vi "WSVCAP SHL FPGA LL Procedure I2C - Send ACK.vi"(0 "Procedure Step":T1, 1 "Wait Ticks Remaining":u32, 5 "I2C Wait Ticks":u32, 7 "ACK Bit to Write":bool, 11 "error in (no error)":errorcluster, 13 "Socket Mask":u64 format="%012x", 14 "UUT (0/1)":u8) -> (3 "Wait Ticks Remaining Out":u32, 4 "Procedure Step Out":T1, 8 "Finished":bool, 15 "error out":errorcluster)   [LabVIEW 2017]
uses:
  Type Defs/WSVCAP SHL Procedure Step Enum.ctl
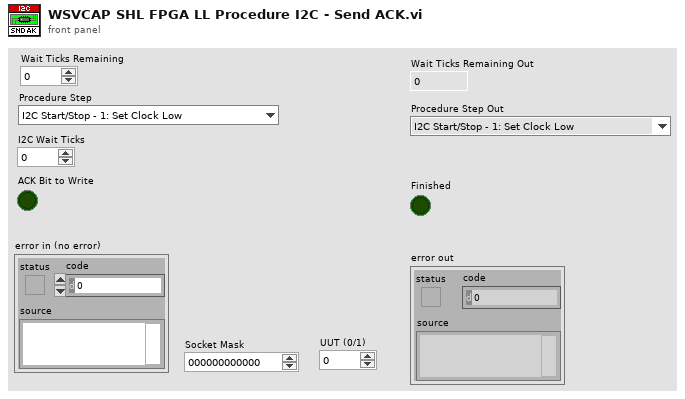
[diagram p1: front panel]
types:
  T1 = typedef "WSVCAP SHL Procedure Step Enum.ctl" = enum16{"I2C Start/Stop - 1: Set Clock Low", "I2C Start/Stop - 2: Wait", "I2C Start/Stop - 3: Set Data I", "I2C Start/Stop - 4: Wait", "I2C Start/Stop - 5: Set Clock High", "I2C Start/Stop - 6: Wait", "I2C Start/Stop - 7: Set Data II", "I2C Start/Stop - 8: Wait", "I2C Start/Stop - 9: Set Clock Low", "I2C Start/Stop - 10: Wait", "I2C Read ACK - 1: Set Clock High", "I2C Read ACK - 2: Wait", "I2C Read ACK - 3: Read ACK Bit", "I2C Read ACK - 4: Wait", "I2C Read ACK - 5: Set Clock Low", "I2C Read ACK - 6: Wait", "I2C Write ACK - 1: Write ACK Bit", "I2C Write ACK - 2: Wait", "I2C Write ACK - 3: Set Clock High", "I2C Write ACK - 4: Wait", "I2C Write ACK - 5: Set Clock Low", "I2C Write ACK - 6: Wait", "I2C Write ACK - 7: Set Data Low", "I2C Send Add - 1: Reset Bits Remaining", "I2C Send Add - 2: Set Data Bit", "I2C Send Add - 3: Wait", "I2C Send Add - 4: Set Clock High", "I2C Send Add - 5: Wait", "I2C Send Add - 6: Set Clock Low", "I2C Send Add - 7: Wait", "I2C Send Add - 8: Check Bits Remaining", "I2C Send Data - 1: Reset Bits Remaining", "I2C Send Data - 2: Load Write Bit from FIFO", "I2C Send Data - 3: Set Data Bit", "I2C Send Data - 4: Wait", "I2C Send Data - 5: Set Clock High", "I2C Send Data - 6: Wait", "I2C Send Data - 7: Set Clock Low", "I2C Send Data - 8: Wait", "I2C Send Data - 9: Check Bits Remaining", "I2C Receive Data - 1: Reset Bits Remaining", "I2C Receive Data - 2: Wait", "I2C Receive Data - 3: Set Clock High", "I2C Receive Data - 4: Wait", "I2C Receive Data - 5: Read Data Bit", "I2C Receive Data - 6: Wait", "I2C Receive Data - 7: Set Clock Low", "I2C Receive Data - 8: Wait", "I2C Receive Data - 9: Check Bits Remaining", "RFFE Send SSC - 1:Set Low", "RFFE Send SSC - 2:Wait", "RFFE Send SSC - 3:Set SDA High", "RFFE Send SSC - 4:Wait", "RFFE Send SSC - 5:Set SDA Low", "RFFE Send SSC - 6:Wait", "RFFE Send Data - 1:Set SCL High", "RFFE Send Data - 2:Wait", "RFFE Send Data - 3:Set SCL Low", "RFFE Send Data - 4:Wait", "RFFE Send Data - 5:Set SCL High (P)", "RFFE Send Data - 6:Wait", "RFFE Send Data - 7:Set SCL Low (P)", "RFFE Send Data - 8:Wait", "RFFE Send Data - 9:Set SCL High (BP)", "RFFE Send Data - 10:Wait", "RFFE Send Data - 11:Set SCL Low (BP)", "RFFE Send Data - 12:Wait", "RFFE Receive Data - 1:Set SCL High", "RFFE Receive Data - 2:Wait", "RFFE Receive Data - 3:Set SCL Low", "RFFE Receive Data - 4:Wait", "RFFE Receive Data - 5:Set SCL High (BP)", "RFFE Receive Data - 6:Wait", "RFFE Receive Data - 7:Set SCL Low (BP)", "RFFE Receive Data - 8:Wait", "RFFE Wait CMD Delay - 1:Wait", "RFFE Clear Lines - 1:Clear"}
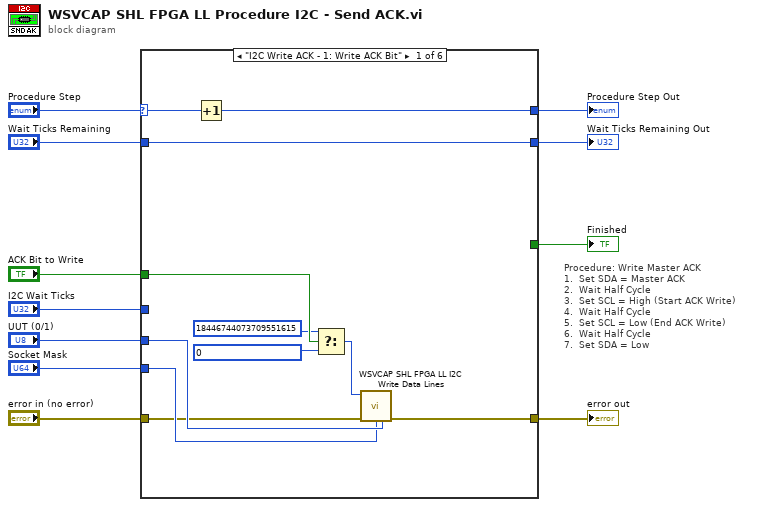
[diagram p0: block diagram]
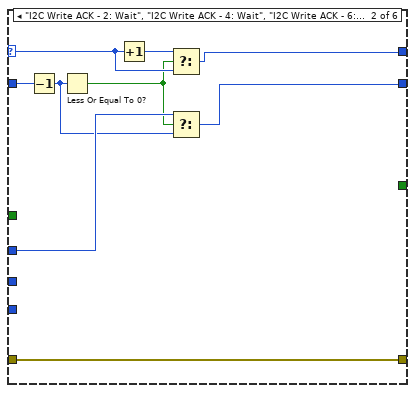
[diagram p2: hidden frame]
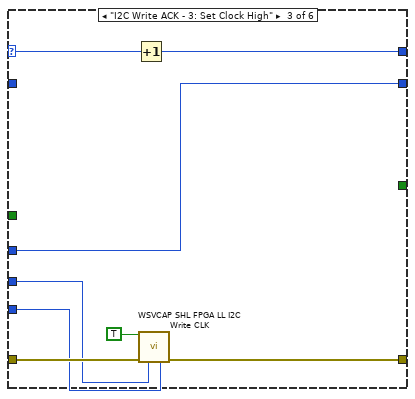
[diagram p3: hidden frame]
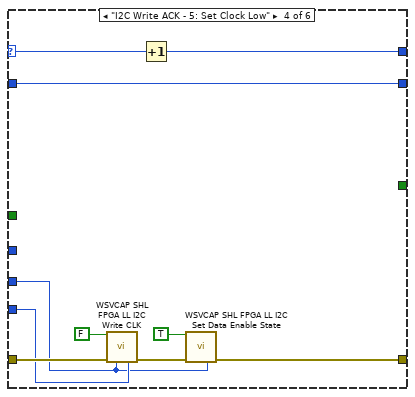
[diagram p4: hidden frame]
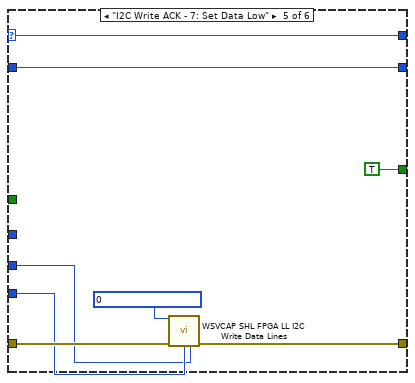
[diagram p5: hidden frame]
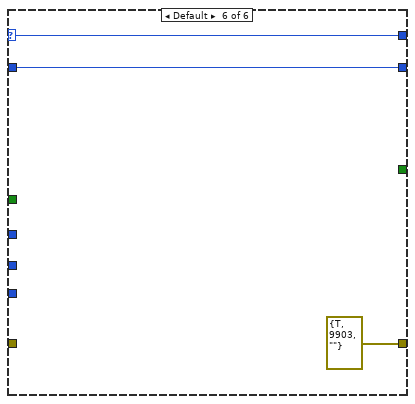
[diagram p6: hidden frame]
diagram:
  # "Procedure: Write Master ACK\n1.  Set SDA = Master ACK\n2.  Wait Half Cycle\n3.  Set SCL = High (Start ACK Write)\n4.  Wait Half Cycle\n5.  Set SCL = Low (End ACK Write)\n6.  Wait Half Cycle\n7.  Set SDA = Low"
  n1 = case shown="\"I2C Write ACK - 1: Write ACK Bit\"" "Procedure Step" {
    selector: "Procedure Step" -> [w22 w26 w37 w44 w56 w59]
    tunnel: [w19 w29 w36 w46 w52 errorcluster {"status"=TRUE, "code"=9903, "source"=""} ("error out")] -> w10
    tunnel: "error in (no error)" -> [w12 w29 w39 w49 w53 _]
    tunnel: "Wait Ticks Remaining" -> [w20 w31 _ w41 w55 w58]
    tunnel: "I2C Wait Ticks" -> [_ w28 w33 _ _ _]
    tunnel: [_ _ _ _ TRUE _] -> w9
    tunnel: "ACK Bit to Write" -> [w18 _ _ _ _ _]
    tunnel: "Socket Mask" -> [w13 _ w35 w43 w51 _]
    tunnel: [w21 w24 w34 w42 w56 w59] -> w3
    tunnel: [w20 w23 w33 w41 w55 w58] -> w2
    tunnel: "UUT (0/1)" -> [w14 _ w32 w40 w50 _]
    frame "I2C Write ACK - 1: Write ACK Bit" {
      n2 = Increment(x=w22) -> (x+1=w21:T1)
      n3 = Select(t=u64 18446744073709551615 ("Write Bit (U64)"), s=w18, f=u64 0 ("Write Bit (U64)")) -> (s? t:f=w15:u64)
      n4 = call "WSVCAP SHL FPGA LL I2C Write Data Lines.vi"("Write Bit (U64)"=w15, "error in (no error)"=w12, "Socket Mask"=w13, "UUT Set (0/1) (Legacy)"=w14) -> ("error out"=w19:errorcluster)  [unwired: 11 in]
    }
    frame "I2C Write ACK - 2: Wait", "I2C Write ACK - 4: Wait", "I2C Write ACK - 6: Wait" {
      n5 = Decrement(x=w31) -> (x-1=w27:u32)
      n6 = Less Or Equal To 0?(x=w27) -> (x <= 0?=w25:bool)
      n7 = Increment(x=w26) -> (x+1=w30:T1)
      n8 = Select(t=w30, s=w25, f=w26) -> (s? t:f=w24:T1)
      n9 = Select(t=w28, s=w25, f=w27) -> (s? t:f=w23:u32)
    }
    frame "I2C Write ACK - 3: Set Clock High" {
      n10 = Increment(x=w37) -> (x+1=w34:T1)
      n11 = call "WSVCAP SHL FPGA LL I2C Write CLK.vi"("Bit In"=TRUE, "error in (no error)"=w39, "UUT Set (0/1 (Legacy)"=w32, "Socket Mask"=w35) -> ("error out"=w36:errorcluster)  [unwired: 11 in]
    }
    frame "I2C Write ACK - 5: Set Clock Low" {
      n12 = call "WSVCAP SHL FPGA LL I2C Write CLK.vi"("Bit In"=FALSE, "error in (no error)"=w49, "UUT Set (0/1 (Legacy)"=w40, "Socket Mask"=w43) -> ("error out"=w47:errorcluster)  [unwired: 11 in]
      n13 = Increment(x=w44) -> (x+1=w42:T1)
      n14 = call "WSVCAP SHL FPGA LL I2C Set Data Enable State.vi"("State"=TRUE, "error in (no error)"=w47, "UUT Set (0/1)"=w40) -> ("error out"=w46:errorcluster)  [unwired: 12 in]
    }
    frame "I2C Write ACK - 7: Set Data Low" {
      n15 = call "WSVCAP SHL FPGA LL I2C Write Data Lines.vi"("Write Bit (U64)"=u64 0, "error in (no error)"=w53, "Socket Mask"=w51, "UUT Set (0/1) (Legacy)"=w50) -> ("error out"=w52:errorcluster)  [unwired: 11 in]
    }
    frame Default {
    }
  }
  "error out" <- w10
  "Finished" <- w9
  "Procedure Step Out" <- w3
  "Wait Ticks Remaining Out" <- w2
